vi "ReadFromFIFOPort4.vi"() -> ()   [LabVIEW 2011]
doc: "Elizabeth Mahon\nJust WriteToFifo backwards, pretty much. Still needs to be tested (as soon as we get the servo controller actually running...)"
uses:
  <vilib>/rvi/eio/common/nirviEmuTemplateMethod_errors.vi
  <vilib>/eio/EIOMethodNode/EIOMethodNode.xnode
panel:
  in  "Data":u8
  in  "StopPort4":bool
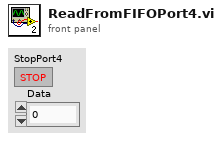
[diagram p1: front panel]
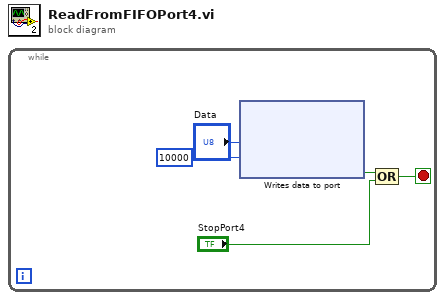
[diagram p0: block diagram]
diagram:
  n1 = while {
    stop <- w4 stop-if-true
    n2 = xnode "Writes data to port"("Data"="Data", "Timeout (ms)"=10000) -> ("Timed Out"=w5:bool)  [unwired: 1 in, 1 out]
    n3 = Compound Arithmetic op=OR(w5, "StopPort4") -> (w4:bool)
  }
